vi "Build Octree from triangles.vi"(3 "Triangle array":T3[](array[typedef]), 4 "World Pmin (x, y, z)":sgl[](array[numeric]), 5 "World Pmax (x, y, z)":sgl[](array[numeric]), 6 "Octree resolution (model units)":sgl) -> (0 "Stack error":errorcluster, 1 "Branch levels":i32, 2 "Octree node array":T1[](array[typedef]))   [LabVIEW 2014]
uses:
  Typedefs/Triangle.ctl
  Typedefs/TreeNodeBox.ctl
  Typedefs/Quad.ctl
panel:
  out "Octree node stack history":i32(graph)
  # "PN 17/01/2015"
  # "Vertices"
  # "Edges"
  # "Unit normal"
  # "Edge unit normals"
  # "Vertices"
  # "Edges"
  # "Unit normal"
  # "Edge unit normals"
  # "Vertices"
  # "Edges"
  # "Unit normal"
  # "Edge unit normals"
  # "Vertices"
  # "Edges"
  # "Unit normal"
  # "Edge unit normals"
  # "Vertices"
  # "Edges"
  # "Unit normal"
  # "Edge unit normals"
  # "Vertices"
  # "Edges"
  # "Unit normal"
  # "Edge unit normals"
  # "Vertices"
  # "Edges"
  # "Unit normal"
  # "pre-store"
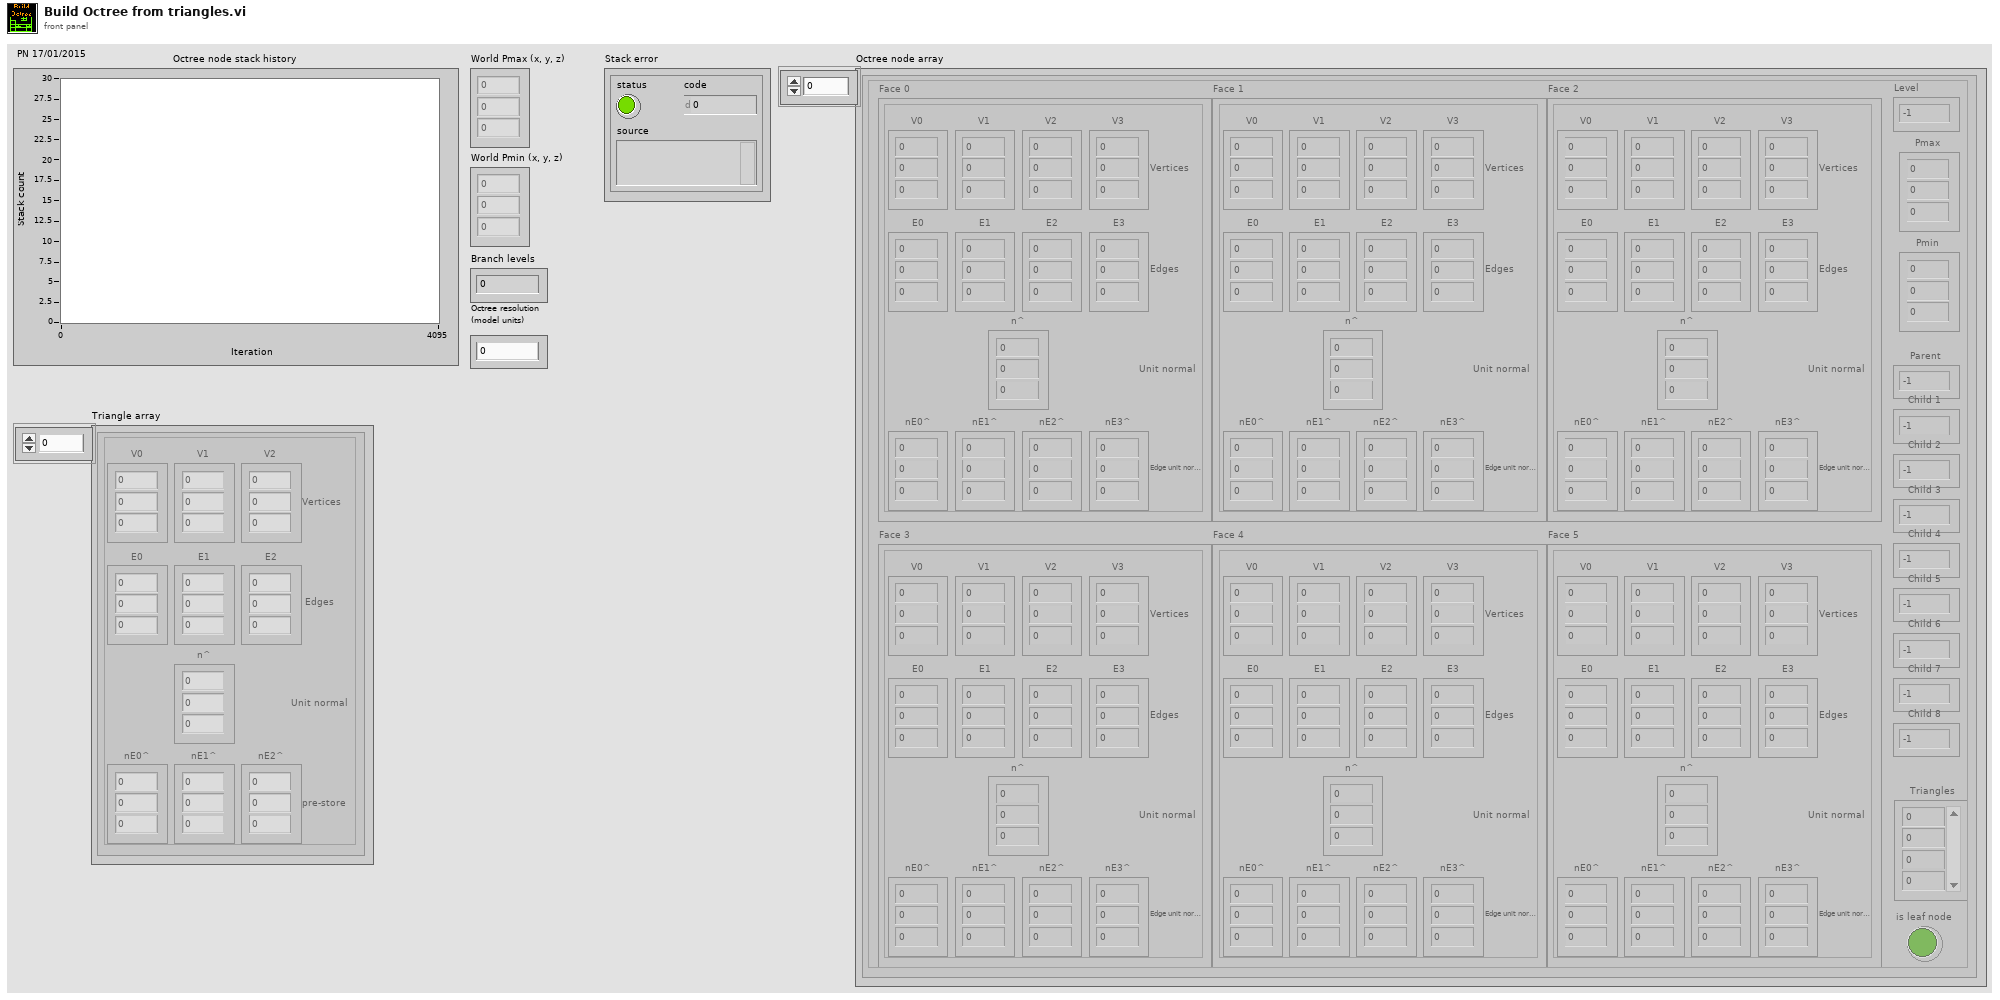
[diagram p1: front panel]
types:
  T1 = typedef "TreeNodeBox.ctl" = cluster{"Face 0":T2, "Face 1":T2, "Face 2":T2, "Face 3":T2, "Face 4":T2, "Face 5":T2, "Level":i32, "Pmax":sgl[], "Pmin":sgl[], "Parent":i32, "Child 1":i32, "Child 2":i32, "Child 3":i32, "Child 4":i32, "Child 5":i32, "Child 6":i32, "Child 7":i32, "Child 8":i32, "Triangles":i32[], "is leaf node":bool}
  T2 = typedef "Quad.ctl" = cluster{"V0":sgl[], "V1":sgl[], "V2":sgl[], "V3":sgl[], "E0":sgl[], "E1":sgl[], "E2":sgl[], "E3":sgl[], "n^":sgl[], "nE0^":sgl[], "nE1^":sgl[], "nE2^":sgl[], "nE3^":sgl[]}
  T3 = typedef "Triangle.ctl" = cluster{"V0":sgl[], "V1":sgl[], "V2":sgl[], "E0":sgl[], "E1":sgl[], "E2":sgl[], "n^":sgl[], "nE0^":sgl[], "nE1^":sgl[], "nE2^":sgl[]}
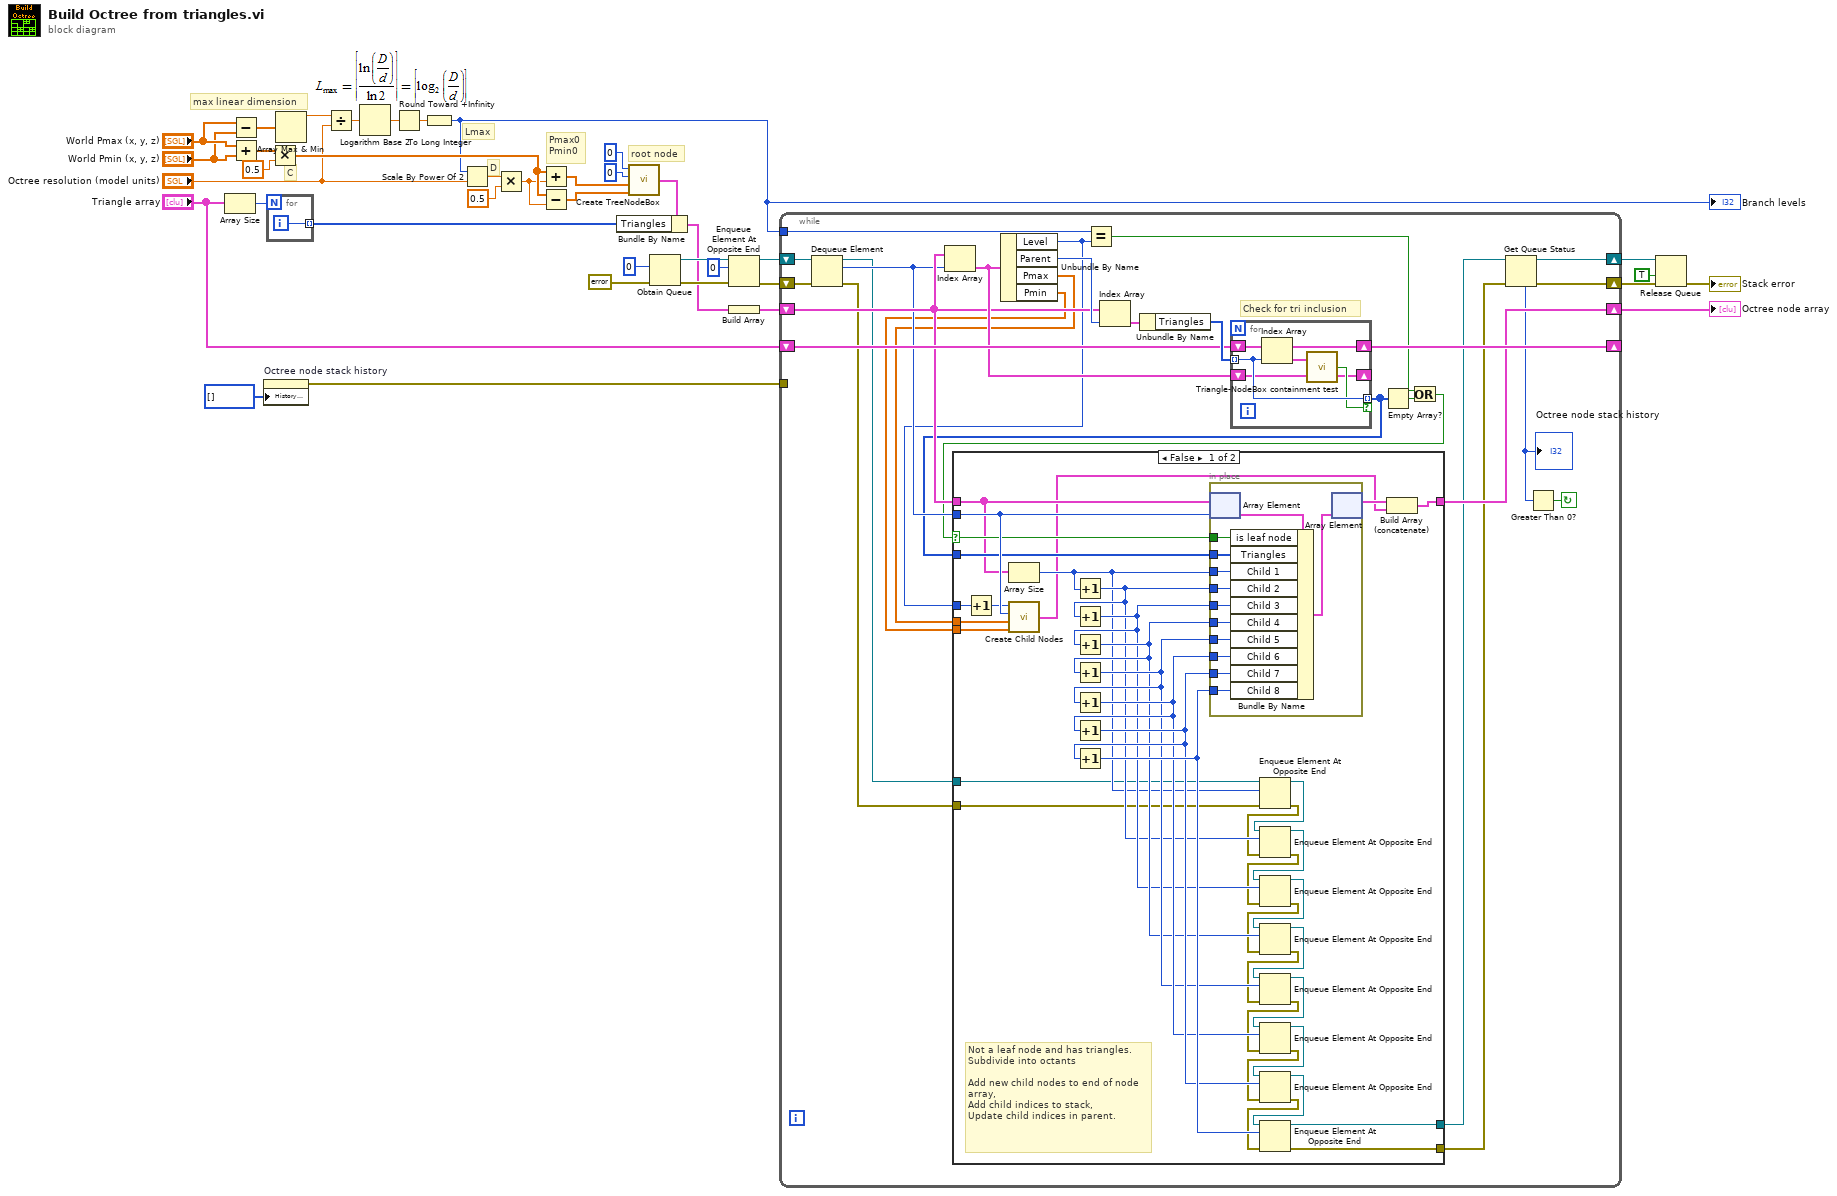
[diagram p0: block diagram]
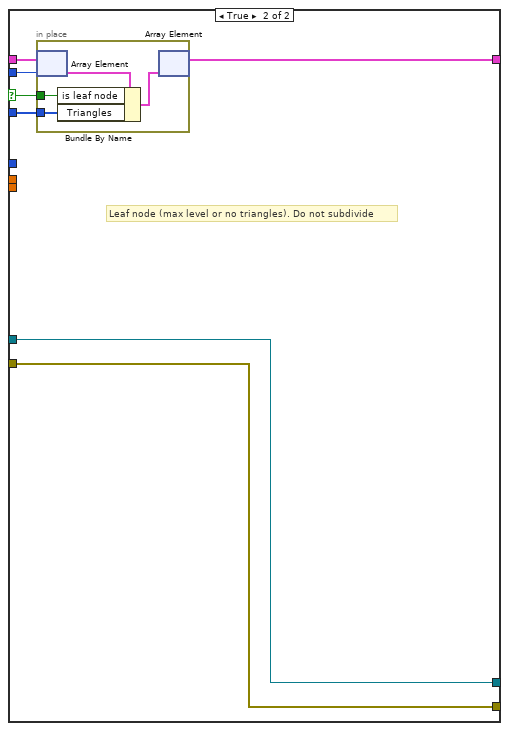
[diagram p2: hidden frame]
diagram:
  # "root node"
  # "D"
  # "Lmax"
  # "Pmax0\nPmin0"
  # "max linear dimension"
  # "C"
  n1 = Array Size(array="Triangle array") -> (size(s)=w19:i32)
  n2 = Subtract(x="World Pmax (x, y, z)", y="World Pmin (x, y, z)") -> (x-y=w35:sgl[])
  n3 = Add(x="World Pmax (x, y, z)", y="World Pmin (x, y, z)") -> (x+y=w39:sgl[])
  n4 = property on="Octree node stack history" class="WFChart (strict)"("History Data"=i32[] []) -> (error out=w3:errorcluster)  [unwired: 2 in, 1 out]
  n5 = for {
    N: w19 -> [_]
    tunnel: [w40] -> w18 mode=indexing
    i -> [w40]
  }
  n6 = Multiply(x=w39, y=sgl 0.5 ("Numeric")) -> (x*y=w33:sgl[])
  n7 = Array Max & Min(array=w35) -> (max value=w31:sgl)  [unwired: 3 out]
  n8 = Divide(x=w31, y="Octree resolution (model units)") -> (x/y=w30:sgl)
  n9 = Logarithm Base 2(1:w30) -> (0:w29:sgl)
  n10 = Round Toward +Infinity(x=w29) -> (ceil(x): smallest int >= x=w28:sgl)
  n11 = To Long Integer(number=w28) -> (32bit integer=w12:i32)
  "Branch levels" <- w12
  n12 = Scale By Power Of 2(n=w12, x="Octree resolution (model units)") -> (x*2^n=w10:sgl)
  n13 = Multiply(x=w10, y=sgl 0.5 ("Numeric")) -> (x*y=w32:sgl)
  n14 = Add(x=w33, y=w32) -> (x+y=w7:sgl[])
  n15 = Subtract(x=w33, y=w32) -> (x-y=w6:sgl[])
  n16 = call "Create TreeNodeBox.vi"("Pmin"=w6, "Pmax"=w7, "Parent"=0, "Level"=0) -> ("Box"=w8:T1)
  n17 = Bundle By Name(cluster=w8, "Triangles"=w18) -> (w17:T1)
  n18 = Obtain Queue(element data type=0, error in (no error)=errorcluster {"status"=FALSE, "code"=0, "source"=""}) -> (queue out=w26:refnum<queue>, error out=w25:errorcluster)  [unwired: 3 in, 1 out]
  n19 = Enqueue Element At Opposite End(queue=w26, element=0, error in (no error)=w25) -> (queue out=w24:refnum<queue>, error out=w23:errorcluster)  [unwired: 1 in, 1 out]
  n20 = Build Array(w17) -> (w16:T1[])
  n21 = while {
    shift-right: [w46] -> w22
    shift-left: w24 -> [w67]
    shift-right: [w64] -> w21
    shift-left: w23 -> [w66]
    shift-right: [w61] -> _
    shift-left: "Triangle array" -> [w62]
    shift-right: [w49] -> w13
    shift-left: w16 -> [w54]
    tunnel: w12 -> [w58]
    tunnel: w3 -> [_]
    stop <- w65 continue-if-true
    # "Check for tri inclusion"
    n22 = Dequeue Element(queue=w67, error in (no error)=w66) -> (queue out=w45:refnum<queue>, element=w53:i32, error out=w44:errorcluster)  [unwired: 1 in, 1 out]
    n23 = Index Array(array=w54, index=w53) -> (element=w55:T1)
    n24 = Unbundle By Name(w55) -> ("Level"=w51:i32, "Parent"=w60:i32, "Pmax"=w47:sgl[], "Pmin"=w48:sgl[])
    n25 = Equal?(x=w58, y=w51) -> (x = y?=w56:bool)
    n26 = Index Array(array=w54, index=w60) -> (element=w59:T1)
    n27 = Unbundle By Name(w59) -> ("Triangles"=w63:i32[])
    n28 = for {
      tunnel: w63 -> [w130] mode=indexing
      shift-right: [w132] -> w61
      shift-left: w62 -> [w132]
      tunnel: [w130] -> w52 mode=indexing if=w129
      shift-right: [w128] -> _
      shift-left: w55 -> [w128]
      n29 = Index Array(array=w132, index=w130) -> (element=w131:T3)
      n30 = call "Triangle-NodeBox containment test.vi"("NodeBox"=w128, "Triangle"=w131) -> ("Triangle is in NodeBox"=w129:bool)
    }
    n31 = Empty Array?(array=w52) -> (empty?=w57:bool)
    n32 = Or(x=w56, y=w57) -> (x .or. y?=w50:bool)
    n33 = case shown="False" w50 {
      selector: w50 -> [w100 w120]
      tunnel: w54 -> [w97 w123]
      tunnel: w53 -> [w104 w122]
      tunnel: w52 -> [w103 w121]
      tunnel: w51 -> [w102 _]
      tunnel: [w96 w119] -> w49
      tunnel: w48 -> [w99 _]
      tunnel: w47 -> [w98 _]
      tunnel: w45 -> [w84 w118]
      tunnel: [w71 w118] -> w43
      tunnel: [w70 w117] -> w42
      tunnel: w44 -> [w69 w117]
      frame False {
        # "Not a leaf node and has triangles.\nSubdivide into octants\n\nAdd new child nodes to end of node array,\nAdd child indices to stack,\nUpdate child indices in parent."
        n34 = Increment(x=w102) -> (x+1=w101:i32)
        n35 = Array Size(array=w97) -> (size(s)=w87:i32)
        n36 = call "Create Child Nodes.vi"("Pmin (parent)"=w99, "Pmax (parent)"=w98, "Parent"=w104, "Level (parent+1)"=w101) -> ("8 Child nodes array"=w68:T1[])
        n37 = Increment(x=w87) -> (x+1=w88:i32)
        n38 = Increment(x=w88) -> (x+1=w89:i32)
        n39 = Increment(x=w89) -> (x+1=w90:i32)
        n40 = Increment(x=w90) -> (x+1=w91:i32)
        n41 = Increment(x=w91) -> (x+1=w92:i32)
        n42 = Increment(x=w92) -> (x+1=w93:i32)
        n43 = Increment(x=w93) -> (x+1=w94:i32)
        n44 = in-place {
          in-place-border: w100 -> [w114]
          in-place-border: w103 -> [w113]
          in-place-border: w87 -> [w112]
          in-place-border: w88 -> [w111]
          in-place-border: w89 -> [w110]
          in-place-border: w90 -> [w109]
          in-place-border: w91 -> [w108]
          in-place-border: w92 -> [w107]
          in-place-border: w93 -> [w106]
          in-place-border: w94 -> [w105]
          n45 = in-place-array #1(w97, w104) -> (w116:T1)
          n46 = Bundle By Name(cluster=w116, "is leaf node"=w114, "Triangles"=w113, "Child 1"=w112, "Child 2"=w111, "Child 3"=w110, "Child 4"=w109, "Child 5"=w108, "Child 6"=w107, "Child 7"=w106, "Child 8"=w105) -> (w115:T1)
          n47 = in-place-array #1(w115) -> (w95:T1[])  [unwired: 1 out]
        }
        n48 = Enqueue Element At Opposite End(queue=w84, element=w87, error in (no error)=w69) -> (queue out=w85:refnum<queue>, error out=w86:errorcluster)  [unwired: 1 in, 1 out]
        n49 = Enqueue Element At Opposite End(queue=w85, element=w88, error in (no error)=w86) -> (queue out=w83:refnum<queue>, error out=w82:errorcluster)  [unwired: 1 in, 1 out]
        n50 = Enqueue Element At Opposite End(queue=w83, element=w89, error in (no error)=w82) -> (queue out=w80:refnum<queue>, error out=w81:errorcluster)  [unwired: 1 in, 1 out]
        n51 = Enqueue Element At Opposite End(queue=w80, element=w90, error in (no error)=w81) -> (queue out=w78:refnum<queue>, error out=w79:errorcluster)  [unwired: 1 in, 1 out]
        n52 = Enqueue Element At Opposite End(queue=w78, element=w91, error in (no error)=w79) -> (queue out=w76:refnum<queue>, error out=w77:errorcluster)  [unwired: 1 in, 1 out]
        n53 = Enqueue Element At Opposite End(queue=w76, element=w92, error in (no error)=w77) -> (queue out=w74:refnum<queue>, error out=w75:errorcluster)  [unwired: 1 in, 1 out]
        n54 = Enqueue Element At Opposite End(queue=w74, element=w93, error in (no error)=w75) -> (queue out=w72:refnum<queue>, error out=w73:errorcluster)  [unwired: 1 in, 1 out]
        n55 = Enqueue Element At Opposite End(queue=w72, element=w94, error in (no error)=w73) -> (queue out=w71:refnum<queue>, error out=w70:errorcluster)  [unwired: 1 in, 1 out]
        n56 = Build Array (concatenate)(w95, w68) -> (w96:T1[])
      }
      frame True {
        # "Leaf node (max level or no triangles). Do not subdivide"
        n57 = in-place {
          in-place-border: w120 -> [w125]
          in-place-border: w121 -> [w124]
          n58 = in-place-array #2(w123, w122) -> (w127:T1)
          n59 = Bundle By Name(cluster=w127, "is leaf node"=w125, "Triangles"=w124) -> (w126:T1)
          n60 = in-place-array #2(w126) -> (w119:T1[])  [unwired: 1 out]
        }
      }
    }
    n61 = Get Queue Status(queue=w43, error in (no error)=w42) -> (queue out=w46:refnum<queue>, error out=w64:errorcluster, # elements in queue=w41:i32)  [unwired: 1 in, 5 out]
    "Octree node stack history" <- w41
    n62 = Greater Than 0?(x=w41) -> (x > 0?=w65:bool)
  }
  "Octree node array" <- w13
  n63 = Release Queue(queue=w22, force destroy? (F)=TRUE, error in (no error)=w21) -> (error out=→"Stack error":errorcluster)  [unwired: 2 out]
